vi "Hide GUI.vi"(7 "Save Pref (T)":bool=TRUE, 8 "error in (no error)":errorcluster, 11 "PluginGUI in":refnum<class "PluginGUI.lvclass">) -> (0 "error out":errorcluster, 3 "PluginGUI out":refnum<class "PluginGUI.lvclass">)   [LabVIEW 2020, in "VolatusGUI.lvlib" / "PluginGUI.lvclass"]
uses:
  PluginGUI.lvclass
  PluginGUI.lvclass/PluginGUI.ctl
  GUI Helper/GUI Helper.lvclass
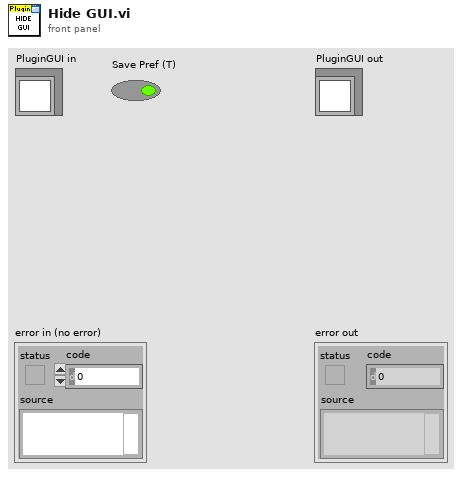
[diagram p1: front panel]
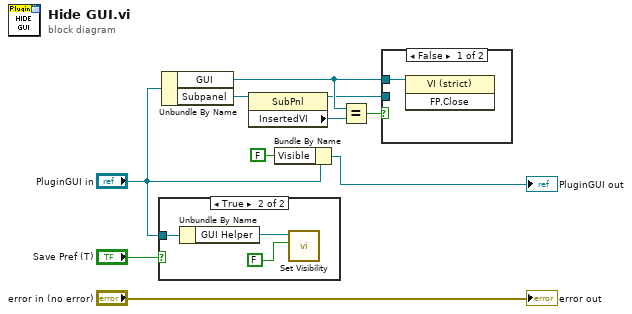
[diagram p0: block diagram]
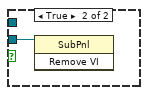
[diagram p3: hidden frame]
diagram:
  n1 = case shown="True" "Save Pref (T)" {
    tunnel: "PluginGUI in" -> [_ w11]
    frame False {
    }
    frame True {
      n2 = Unbundle By Name(w11) -> ("GUI Helper"=w13:refnum<class "MessageQ.lvclass">)
      n3 = call "Set Visibility.vi"("Visible"=FALSE, "GUI Helper in"=w13) -> ()  [unwired: 8 in, 2 out]
    }
  }
  n4 = Unbundle By Name("PluginGUI in") -> ("GUI"=w8:refnum<vi>, "Subpanel"=w10:refnum<vi>)
  n5 = property class="SubPnl"(reference=w10) -> (reference out=w6:refnum<vi>, "InsertedVI"=w9:refnum<vi>)  [unwired: 1 in, 1 out]
  n6 = Bundle By Name(cluster="PluginGUI in", "Visible"=FALSE) -> (→"PluginGUI out":refnum<class "PluginGUI.lvclass">)
  n7 = Equal?(x=w8, y=w9) -> (x = y?=w7:bool)
  n8 = case shown="False" w7 {
    tunnel: w8 -> [w14 _]
    tunnel: w6 -> [_ w15]
    frame False {
      n9 = invoke class="VI (strict)" method="FP.Close"(reference=w14) -> ()  [unwired: 2 in, 3 out]
    }
    frame True {
      n10 = invoke class="SubPnl" method="Remove VI"(reference=w15) -> ()  [unwired: 2 in, 3 out]
    }
  }
  "error out" <- "error in (no error)"
